vi "Drop.vi"(8 "error in (no error)":errorcluster, 11 "OrderSelection in":refnum<class "OrderSelection.lvclass">) -> (0 "error out":errorcluster, 3 "OrderSelection out":refnum<class "OrderSelection.lvclass">)   [LabVIEW 2020, in "OrderSelection.lvclass"]
uses:
  OrderSelection.lvclass
  C:/Program Files/National Instruments/LabVIEW 2020/vi.lib/QSI/QControls/QControl Classes/Control/Control.lvclass
  Read Items.vi
  Read SelectedItem.vi
  Read PositionIndex.vi
  Write SelectedItem.vi
  Write Items.vi
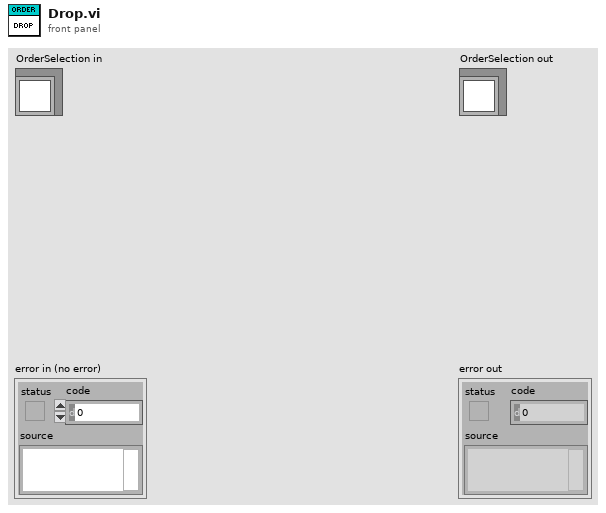
[diagram p1: front panel]
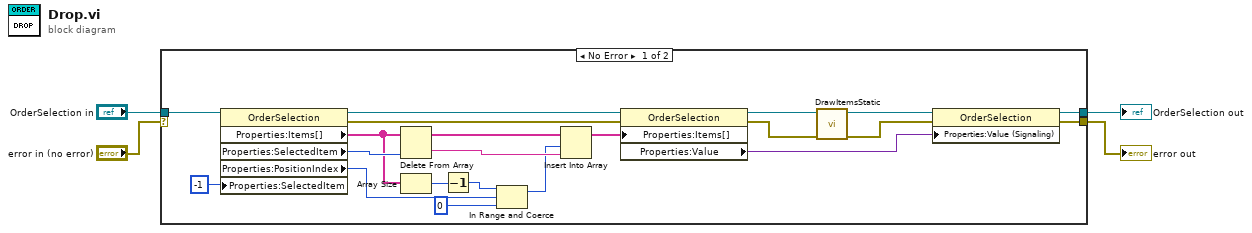
[diagram p0: block diagram]
diagram:
  n1 = case shown="No Error" "error in (no error)" {
    selector: "error in (no error)" -> [_ w27]
    tunnel: [w14 w27] -> w3
    tunnel: [w12 w26] -> w1
    tunnel: "OrderSelection in" -> [w25 w26]
    frame No Error {
      n2 = property class="OrderSelection"(reference=w25, "Properties:SelectedItem"=-1 ("SelectedItem")) -> (reference out=w19:refnum<class "OrderSelection.lvclass">, error out=w24:errorcluster, "Properties:Items[]"=w9:string[], "Properties:SelectedItem"=w22:i32, "Properties:PositionIndex"=w10:i32)  [unwired: 1 in]
      n3 = Delete From Array(array=w9, index=w22) -> (deleted portion=w20:string, array with subset deleted=w21:string[])  [unwired: 1 in]
      n4 = Array Size(array=w9) -> (size(s)=w8:i32)
      n5 = Decrement(x=w8) -> (x-1=w5:i32)
      n6 = In Range and Coerce(upper limit=w5, x=w10, lower limit=0) -> (coerced(x)=w6:i32)  [unwired: 1 out]
      n7 = Insert Into Array(array=w21, index=w6, new element=w20) -> (w18:string[])
      n8 = property class="OrderSelection"(reference=w19, error in=w24, "Properties:Items[]"=w18) -> (reference out=w17:refnum<class "OrderSelection.lvclass">, error out=w16:errorcluster, "Properties:Value"=w11:variant)
      n9 = call "DrawItemsStatic.vi"("error in (no error)"=w16, "OrderSelection in"=w17) -> ("error out"=w15:errorcluster, "OrderSelection out"=w13:refnum<class "OrderSelection.lvclass">)  [unwired: 8 in]
      n10 = property class="OrderSelection"(reference=w13, error in=w15, "Properties:Value (Signaling)"=w11) -> (reference out=w12:refnum<class "OrderSelection.lvclass">, error out=w14:errorcluster)
    }
    frame Error {
    }
  }
  "error out" <- w3
  "OrderSelection out" <- w1
